vi "HIOKI PW3390 Conf Motor Common.vi"(0 "VISA Resource":refnum<visa-resource-name>, 1 "Set/Query (F: Set)":bool, 5 "Sync Source (9: DC50m)":T1(ring)=enum."DC50ms", 7 "LPF (0: OFF)":enum16{"OFF", "ON"}(ring), 9 "Slip (0: f1)":enum16{"f1", "f2", "f3", "f4"}(ring), 11 "error in (no error)":errorcluster, 12 "OPC query (T: ON)":bool=TRUE, 13 "Error Out (F: Off)":bool) -> (4 "VISA Resource out":refnum<visa-resource-name>, 6 "Sync Source out":T1(ring)=enum."DC50ms", 8 "LPF out":enum16{"OFF", "ON"}(ring), 10 "Slip out":enum16{"f1", "f2", "f3", "f4"}(ring), 15 "error out":errorcluster)   [LabVIEW 2009]
doc: "Sets and reads the functions related to the Motor Analysis Option's both Channel A and B.\n\nSet/Query\n Set: Send the setting commands for the device.\n Query: Query the setting of the device.\n\nSync Source\n Sets the motor synchronized source.\n\nLPF\n Sets the low pass filter for the motor analysis.\n\nSlip\n Sets the frequency source for the slip calculation."
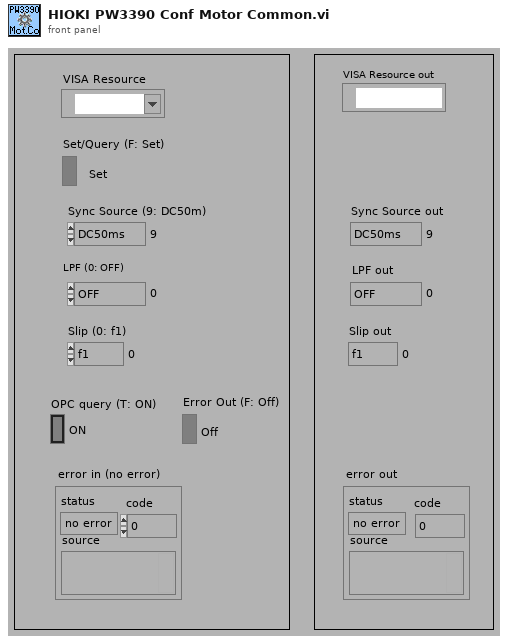
[diagram p1: front panel]
types:
  T1 = enum16{"U1", "U2", "U3", "U4", "I1", "I2", "I3", "I4", "Ext", "DC50ms", "DC100ms"}
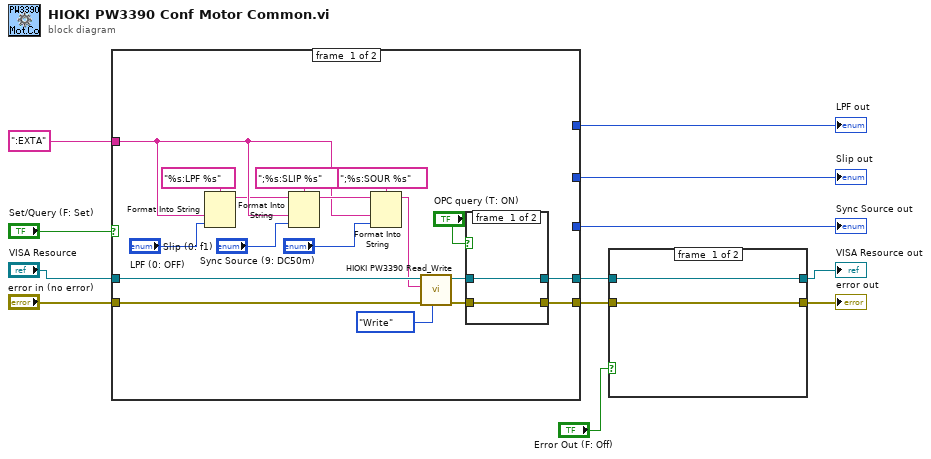
[diagram p0: block diagram]
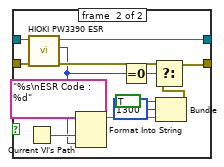
[diagram p2: hidden frame]
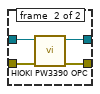
[diagram p3: hidden frame]
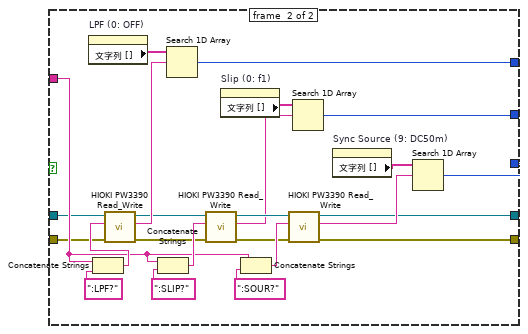
[diagram p4: hidden frame]
diagram:
  n1 = case shown="FALSE" "Set/Query (F: Set)" {
    tunnel: "error in (no error)" -> [w27 w45]
    tunnel: [w15 w37] -> w4
    tunnel: "VISA Resource" -> [w28 w44]
    tunnel: [w16 w38] -> w5
    tunnel: ":EXTA" -> [w20 w46]
    tunnel: [_ w52] -> w9
    tunnel: [_ w51] -> w8
    tunnel: [_ w41] -> w7
    frame #0 {
      n2 = Format Into String(format string="%s:LPF %s", w20, "LPF (0: OFF)") -> (resulting string=w14:string)  [unwired: 2 in, 1 out]
      n3 = Format Into String(format string=";%s:SLIP %s", initial string=w14, w20, "Slip (0: f1)") -> (resulting string=w24:string)  [unwired: 1 in, 1 out]
      n4 = Format Into String(format string=";%s:SOUR %s", initial string=w24, w20, "Sync Source (9: DC50m)") -> (resulting string=w13:string)  [unwired: 1 in, 1 out]
      n5 = call <instrlib>:"HIOKI PW3390 Read_Write.vi"("Read/Write"=enum16{"Read", "Write"}."Write", "error in (no error)"=w27, "data in"=w13, "VISA Resource"=w28) -> ("error out"=w17:errorcluster, "VISA Resource out"=w18:refnum<visa-resource-name>)  [unwired: 5 in, 1 out]
      n6 = case shown="TRUE" "OPC query (T: ON)" {
        tunnel: [w32 w36] -> w16
        tunnel: [w31 w35] -> w15
        tunnel: w18 -> [w32 w34]
        tunnel: w17 -> [w31 w33]
        frame #0 {
        }
        frame #1 {
          n7 = call <instrlib>:"HIOKI PW3390 OPC.vi"("error in (no error)"=w33, "VISA Resource"=w34) -> ("error out"=w35:errorcluster, "VISA Resource out"=w36:refnum<visa-resource-name>)  [unwired: 7 in, 1 out]
        }
      }
    }
    frame #1 {
      n8 = property on="LPF (0: OFF)" class="Enum (strict)"() -> ("文字列 []"=w43:string[])  [unwired: 2 in, 2 out]
      n9 = Concatenate Strings(w46, ":LPF?") -> (w48:string)
      n10 = call <instrlib>:"HIOKI PW3390 Read_Write.vi"("error in (no error)"=w45, "data in"=w48, "VISA Resource"=w44) -> ("error out"=w39:errorcluster, "data out"=w42:string, "VISA Resource out"=w40:refnum<visa-resource-name>)  [unwired: 6 in]
      n11 = Concatenate Strings(w46, ":SLIP?") -> (w60:string)
      n12 = Search 1D Array(1D array=w43, element=w42) -> (index of element=w41:i32)  [unwired: 1 in]
      n13 = call <instrlib>:"HIOKI PW3390 Read_Write.vi"("error in (no error)"=w39, "data in"=w60, "VISA Resource"=w40) -> ("error out"=w56:errorcluster, "data out"=w49:string, "VISA Resource out"=w55:refnum<visa-resource-name>)  [unwired: 6 in]
      n14 = property on="Slip (0: f1)" class="Enum (strict)"() -> ("文字列 []"=w54:string[])  [unwired: 2 in, 2 out]
      n15 = Concatenate Strings(w46, ":SOUR?") -> (w57:string)
      n16 = call <instrlib>:"HIOKI PW3390 Read_Write.vi"("error in (no error)"=w56, "data in"=w57, "VISA Resource"=w55) -> ("error out"=w37:errorcluster, "data out"=w50:string, "VISA Resource out"=w38:refnum<visa-resource-name>)  [unwired: 6 in]
      n17 = Search 1D Array(1D array=w54, element=w49) -> (index of element=w52:i32)  [unwired: 1 in]
      n18 = property on="Sync Source (9: DC50m)" class="Enum (strict)"() -> ("文字列 []"=w53:string[])  [unwired: 2 in, 2 out]
      n19 = Search 1D Array(1D array=w53, element=w50) -> (index of element=w51:i32)  [unwired: 1 in]
    }
  }
  "Sync Source out" <- w8
  "Slip out" <- w9
  "LPF out" <- w7
  n20 = case shown="TRUE" "Error Out (F: Off)" {
    tunnel: w5 -> [w62 w75]
    tunnel: w4 -> [w61 w74]
    tunnel: [w61 w64] -> w3
    tunnel: [w62 w73] -> w1
    frame #0 {
    }
    frame #1 {
      n21 = Current VI's Path() -> (path=w71:path)
      n22 = call <instrlib>:"HIOKI PW3390 ESR.vi"("error in (no error)"=w74, "VISA Resource"=w75) -> ("error out"=w65:errorcluster, "Output Value"=w63:u8, "VISA Resource out"=w73:refnum<visa-resource-name>)  [unwired: 6 in, 1 out]
      n23 = Format Into String(format string="%s\nESR Code : %d", w71, w63) -> (resulting string=w67:string)  [unwired: 2 in, 1 out]
      n24 = Equal To 0?(x=w63) -> (x = 0?=w72:bool)
      n25 = Bundle("status"=TRUE, "code"=1300, w67) -> (w66:cluster{"status":bool, "code":i32, string})  [unwired: 1 in]
      n26 = Select(t=w65, s=w72, f=w66) -> (s? t:f=w64:errorcluster)
    }
  }
  "error out" <- w3
  "VISA Resource out" <- w1
